vi "Rename Channel.vi"(8 "error in (no error)":errorcluster, 9 "Index":i32, 10 "Name":string, 11 "SignalManager in":refnum<class "SignalManager.lvclass">) -> (0 "error out":errorcluster, 2 "Old name":string, 3 "SignalManager out":refnum<class "SignalManager.lvclass">)   [LabVIEW 2015, in "SignalManager.lvclass"]
uses:
  SignalManager.lvclass
  SignalManager.lvclass/SignalManager.ctl
  Channel/Channel.lvclass/Channel.ctl
  Channel/Read Name.vi
  Channel/Write Name.vi
  Channel/Channel.lvclass
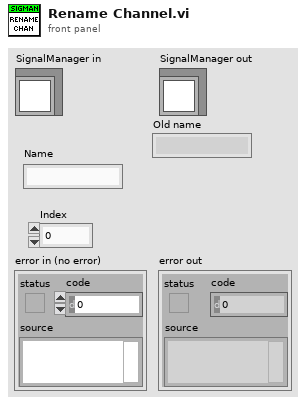
[diagram p1: front panel]
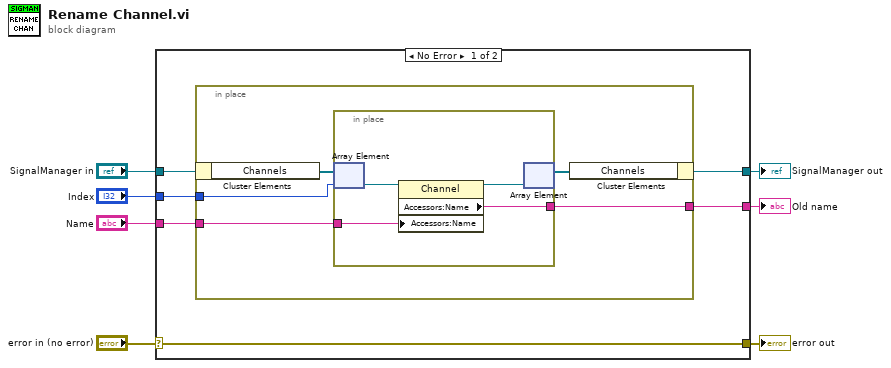
[diagram p0: block diagram]
diagram:
  n1 = case shown="No Error" "error in (no error)" {
    selector: "error in (no error)" -> [w13 w24]
    tunnel: [w13 w24] -> w6
    tunnel: [w11 w23] -> w4
    tunnel: "SignalManager in" -> [w12 w23]
    tunnel: "Index" -> [w10 _]
    tunnel: "Name" -> [w9 _]
    tunnel: [w8 _] -> w1
    frame No Error {
      n2 = in-place {
        in-place-border: w10 -> [w17]
        in-place-border: w9 -> [w16]
        in-place-border: [w14] -> w8
        n3 = in-place-cluster #1(w12) -> ("Channels"=w18:refnum<class "Channel.lvclass">[])
        n4 = in-place {
          in-place-border: w16 -> [w20]
          in-place-border: [w19] -> w14
          n5 = in-place-array #2(w18, w17) -> (w22:refnum<class "Channel.lvclass">)
          n6 = property class="Channel"(reference=w22, "Accessors:Name"=w20) -> (reference out=w21:refnum<class "Channel.lvclass">, "Accessors:Name"=w19:string)  [unwired: 1 in, 1 out]
          n7 = in-place-array #2(w21) -> (w15:refnum<class "Channel.lvclass">[])  [unwired: 1 out]
        }
        n8 = in-place-cluster #1("Channels"=w15) -> (w11:refnum<class "SignalManager.lvclass">)
      }
    }
    frame Error {
    }
  }
  "error out" <- w6
  "SignalManager out" <- w4
  "Old name" <- w1
